vi "Write Simple Address.vi"(8 "error in (no error)":errorcluster, 10 "Simple Address":i32, 11 "Simple Tree Queue Mailman in":refnum<class "Simple Tree Queue Mailman.lvclass">) -> (0 "error out":errorcluster, 3 "Simple Tree Queue Mailman out":refnum<class "Simple Tree Queue Mailman.lvclass">)   [LabVIEW 2024, in "Simple Tree Queue Mailman.lvclass"]
uses:
  Simple Tree Queue Mailman.lvclass
  Simple Tree Queue Mailman.lvclass/Simple Tree Queue Mailman.ctl
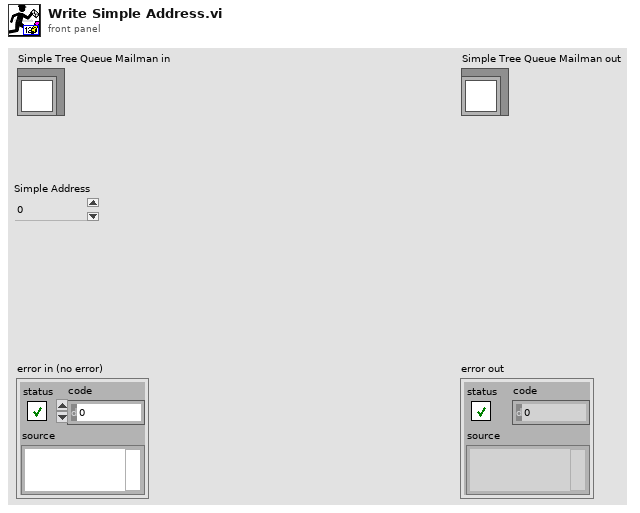
[diagram p1: front panel]
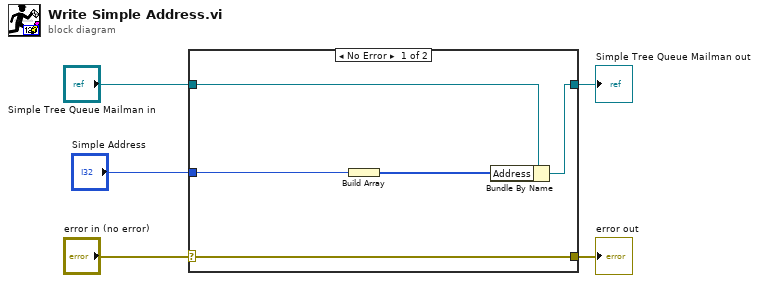
[diagram p0: block diagram]
diagram:
  n1 = case shown="No Error" "error in (no error)" {
    selector: "error in (no error)" -> [w10 w11]
    tunnel: [w10 w11] -> w4
    tunnel: [w8 w12] -> w2
    tunnel: "Simple Tree Queue Mailman in" -> [w9 w12]
    tunnel: "Simple Address" -> [w7 _]
    frame No Error {
      n2 = Build Array(w7) -> (w6:i32[])
      n3 = Bundle By Name(cluster=w9, "Address"=w6) -> (w8:refnum<class "Simple Tree Queue Mailman.lvclass">)
    }
    frame Error {
    }
  }
  "error out" <- w4
  "Simple Tree Queue Mailman out" <- w2
